vi "UsrProfiles-Add user.vi"   [LabVIEW 2017]
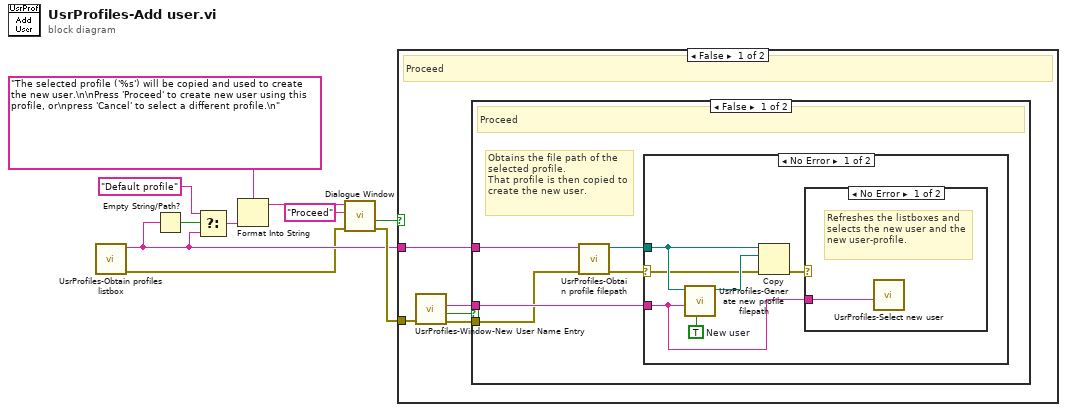
[diagram p0: block diagram]
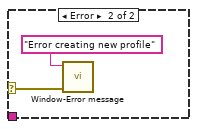
[diagram p2: hidden frame]
diagram:
  n1 = call "UsrProfiles-Obtain profiles listbox.vi"() -> ("error out"=w1:errorcluster, "Selected profile's name"=w2:string)  [unwired: 8 in, 2 out]
  n2 = Empty String/Path?(string/path=w2) -> (empty?=w9:bool)
  n3 = Select(t="Default profile", s=w9, f=w2) -> (s? t:f=w7:string)
  n4 = Format Into String(format string="The selected profile ('%s') will be copied and used to create the new user.\n\nPress 'Proceed' to create new user using this profile, or\npress 'Cancel' to select a different profile.\n" ("Message string"), w7) -> (resulting string=w6:string)  [unwired: 2 in, 1 out]
  n5 = call "Dialogue Window.vi"("error in (no error)"=w1, "Caption-Right button (OK)"="Proceed", "Message string"=w6) -> ("error out"=w3:errorcluster, "Cancelled (Left button pressed)"=w4:bool)  [unwired: 6 in, 1 out]
  n6 = case shown="False" w4 {
    tunnel: w2 -> [w15 _]
    tunnel: w3 -> [w13 _]
    frame False {
      # "Proceed"
      n7 = call "UsrProfiles-Window-New User Name Entry.vi"("error in (no error)"=w13) -> ("error out"=w12:errorcluster, "Cancelled (Left button pressed)"=w14:bool, "New user name"=w11:string)  [unwired: 8 in]
      n8 = case shown="False" w14 {
        tunnel: w15 -> [w20 _]
        tunnel: w11 -> [w19 _]
        tunnel: w12 -> [w17 _]
        frame False {
          # "Obtains the file path of the selected profile.\nThat profile is then copied to create the new user."
          # "Proceed"
          n9 = call "UsrProfiles-Obtain profile filepath.vi"("error in"=w17, "Profile name"=w20) -> ("error out"=w18:errorcluster, "Profile filepath"=w16:path)  [unwired: 8 in]
          n10 = case shown="No Error" w18 {
            selector: w18 -> [w23 _]
            tunnel: w19 -> [w22 _]
            tunnel: w16 -> [w26 _]
            frame No Error {
              w21 = TRUE  # New user
              n11 = call "UsrProfiles-Generate new profile filepath.vi"("New user"=w21, "Destination User name"=w22, "Copied profile's filepath"=w26) -> ("Filepath of profile to be created"=w25:path)  [unwired: 8 in]
              n12 = Copy(8:w23, 10:w25, 11:w26) -> (0:w24:errorcluster)  [unwired: 2 in, 2 out]
              n13 = case shown="No Error" w24 {
                selector: w24 -> [_ w28]
                tunnel: w22 -> [w27 _]
                frame No Error {
                  # "Refreshes the listboxes and selects the new user and the new user-profile."
                  n14 = call "UsrProfiles-Select new user.vi"("New user name"=w27) -> ()  [unwired: 11 in]
                }
                frame Error {
                  n15 = call "Window-Error message.vi"("error in (no error)"=w28, "Message"="Error creating new profile") -> ()  [unwired: 9 in, 1 out]
                }
              }
            }
            frame Error {
            }
          }
        }
        frame True {
          # "Cancelled"
        }
      }
    }
    frame True {
      # "Cancelled"
    }
  }
